vi "testAttitude.vi"() -> ()   [LabVIEW 2011]
uses:
  Instance           3 20Saved   testAttitude .vi
  Instance           1 20Saved   testAttitude .vi
  Instance           2 20Saved   testAttitude .vi
  sbgLabView/sbgLabView.lvlib
panel:
  out "triggerMask":string
  out "XY Graph":cluster{"Y":dbl[], "Y":dbl[]}[](graph)
  out "yaw":sgl format="%#.2f"
  out "pitch":sgl format="%#.2f"
  out "roll":sgl format="%#.2f"
  in  "stop main loop":bool
  in  "Com Port":string
  in  "BaudRate":dbl
  # "sbgLabView Example, Display euler angles for IG devices, Version 1.1"
  # "Copyright (C) SBG Systems 2007-2012 - All right reserved."
  # "www.sbg-systems.com"
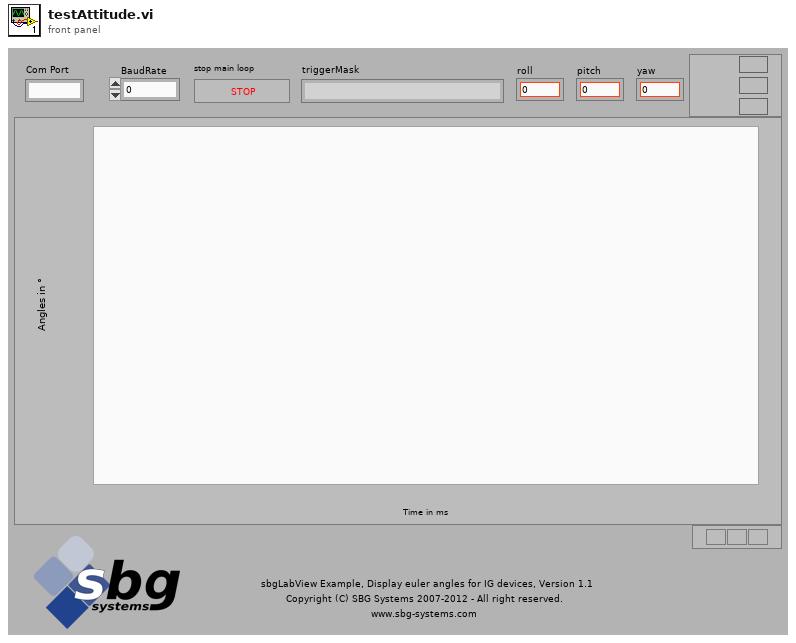
[diagram p1: front panel]
types:
  T1 = cluster{"q0":sgl, "q1":sgl, "q2":sgl, "q3":sgl, "roll":sgl, "pitch":sgl, "yaw":sgl, "ma0":sgl, "ma1":sgl, "ma2":sgl, "ma3":sgl, "ma4":sgl, "ma5":sgl, "ma6":sgl, "ma7":sgl, "ma8":sgl, "g0":sgl, "g1":sgl, "g2":sgl, "a0":sgl, "a1":sgl, "a2":sgl, "m0":sgl, "m1":sgl, "m2":sgl, "t0":sgl, "t1":sgl, "gT0":sgl, "gT1":sgl, "gT2":sgl, "gR0":u16, "gR1":u16, "gR2":u16, "aR0":u16, "aR1":u16, "aR2":u16, "mR0":u16, "mR1":u16, "mR2":u16, "tR0":u16, "tR1":u16, "gTR0":u16, "gTR1":u16, "gTR2":u16, "timeSinceReset":u32, "deviceStatus":sgl, "@dummy control@":u32, "gpsLatitude":dbl, "gpsLongitude":dbl, "gpsAltitude":i32, "gpsV0":i32, "gpsV1":i32, "gpsV2":i32, "gpsHeading":sgl, "gpsHorAccuracy":u32, "gpsVertAccuracy":u32, "gpsSpeedAccuracy":u32, "gpsHeadingAccuracy":sgl, "gpsTimeMs":u32, "gpsFlags":u8, "gpsNbSats":u8, "@dummy control@":u16, "gpsTrueHeading":sgl, "gpsTrueHeadingAccuracy":sgl, "baroPressure":sgl, "baroAltitude":sgl, "@dummy control@":u32, "p0":dbl, "p1":dbl, "p2":dbl, "v0":sgl, "v1":sgl, "v2":sgl, "attitudeAccuracy":sgl, "positionAccuracy":sgl, "velocityAccuracy":sgl, "utcYear":u8, "utcMonth":sgl, "utcDay":sgl, "utcHour":sgl, "utcMin":sgl, "utcSec":u8, "@dummy control@":u16, "utcNano":u32, "magCalibData0":u32, "magCalibData1":u32, "magCalibData2":u32, "odoRawVel0":sgl, "odoRawVel1":sgl, "deltaAngleX":sgl, "deltaAngleY":sgl, "deltaAngleZ":sgl, "heave":sgl}
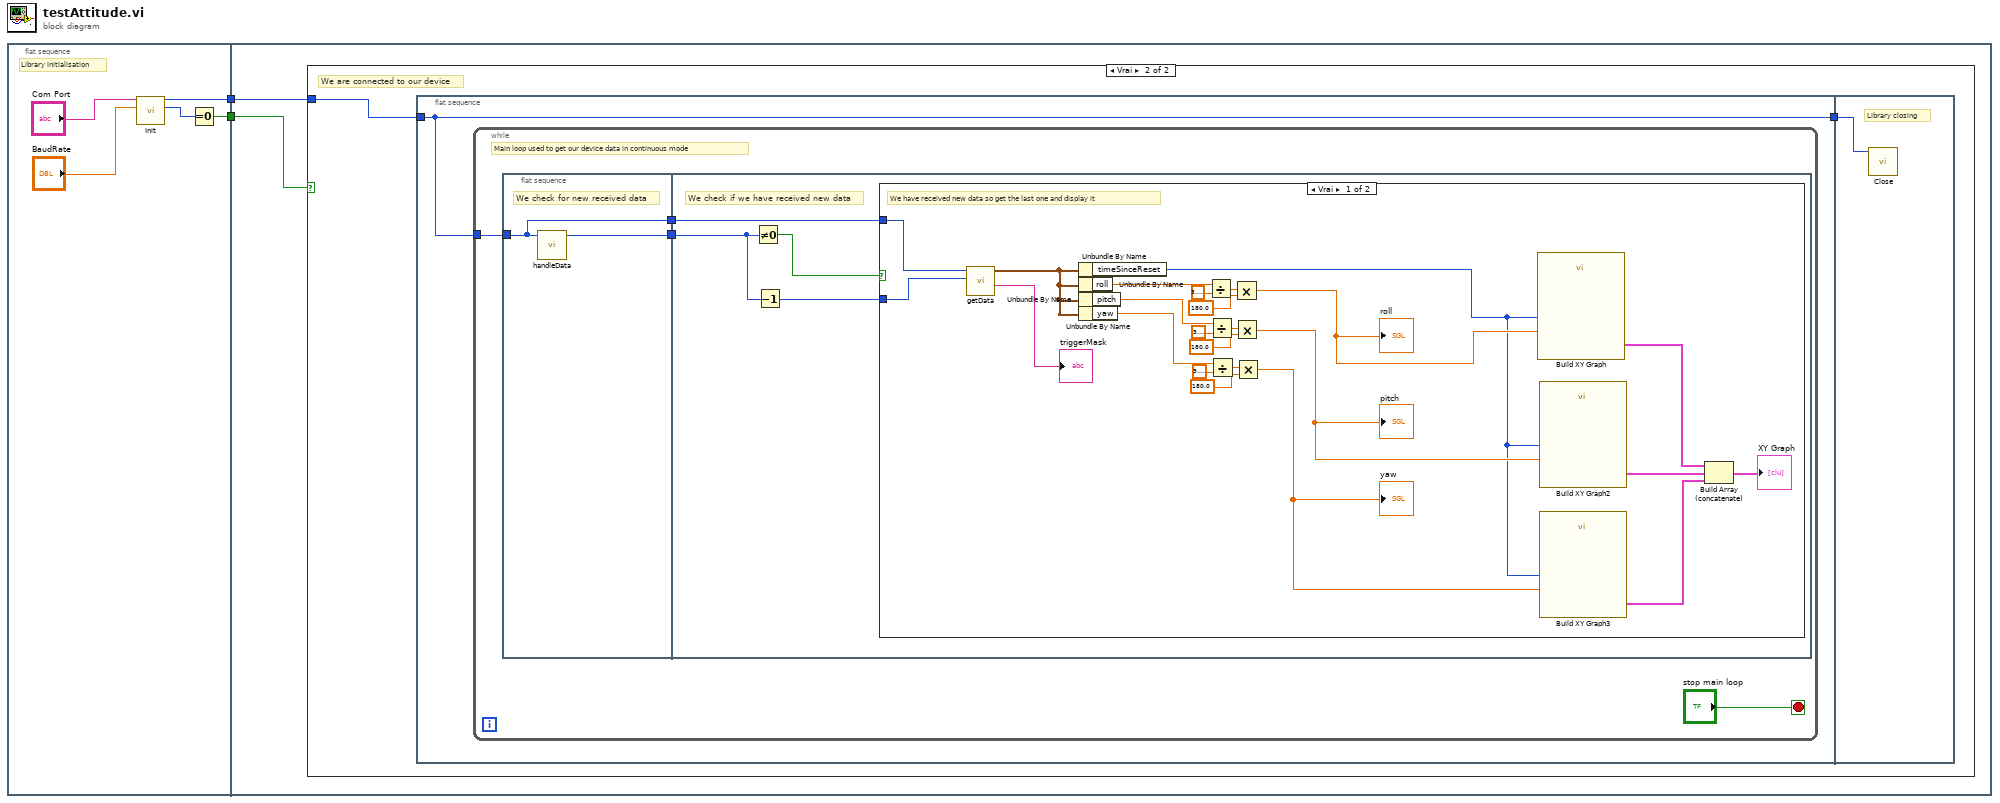
[diagram p0: block diagram]
diagram:
  n1 = flat-sequence {
    tunnel: [w5] -> w2
    tunnel: [w3] -> w1
    tunnel: w2 -> [w8]
    tunnel: w1 -> [w9]
    frame #0 {
      # "Library initialisation"
      n2 = call "Init.vi"("baudRate"="BaudRate", "deviceName"="Com Port") -> ("return type"=w4:i32, "pHandle"=w5:u32)  [unwired: 7 in, 1 out]
      n3 = Equal To 0?(x=w4) -> (x = 0?=w3:bool)
    }
    frame #1 {
      n4 = case shown="Vrai" w9 {
        tunnel: w8 -> [_ w11]
        frame False {
          # "We are not connected to our device"
        }
        frame True {
          # "We are connected to our device"
          n5 = flat-sequence {
            tunnel: w11 -> [w12]
            tunnel: [w12] -> w10
            tunnel: w10 -> [w47]
            frame #0 {
              n6 = while {
                tunnel: w12 -> [w16]
                stop <- "stop main loop" stop-if-true
                # "Main loop used to get our device data in continuous mode"
                n7 = flat-sequence {
                  tunnel: w16 -> [w17]
                  tunnel: [w18] -> w14
                  tunnel: [w17] -> w13
                  tunnel: w14 -> [w21]
                  tunnel: w13 -> [w19]
                  frame #0 {
                    # "We check for new received data"
                    n8 = call "handleData.vi"("pHandle"=w17) -> ("pNumData"=w18:u32)  [unwired: 8 in, 2 out]
                  }
                  frame #1 {
                    # "We check if we have received new data"
                    n9 = Not Equal To 0?(x=w21) -> (x != 0?=w22:bool)
                    n10 = Decrement(x=w21) -> (x-1=w20:u32)
                    n11 = case shown="Vrai" w22 {
                      tunnel: w20 -> [w26 _]
                      tunnel: w19 -> [w25 _]
                      frame True {
                        # "We have received new data so get the last one and display it"
                        n12 = call "getData.vi"("index"=w26, "pHandle"=w25) -> ("triggerMask"=→"triggerMask":string, "pData"=w46:T1)  [unwired: 6 in, 2 out]
                        n13 = Unbundle By Name(w46) -> ("timeSinceReset"=w24:u32)
                        n14 = Unbundle By Name(w46) -> ("roll"=w39:sgl)
                        n15 = Unbundle By Name(w46) -> ("pitch"=w31:sgl)
                        n16 = Unbundle By Name(w46) -> ("yaw"=w30:sgl)
                        n17 = Divide(x=w39, y=3.141592653589793) -> (x/y=w41:dbl)
                        n18 = Divide(x=w31, y=3.141592653589793) -> (x/y=w37:dbl)
                        n19 = Divide(x=w30, y=3.141592653589793) -> (x/y=w34:dbl)
                        n20 = Multiply(x=w41, y=180.0) -> (x*y=w29:dbl)
                        "roll" <- w29
                        n21 = Multiply(x=w37, y=180.0) -> (x*y=w28:dbl)
                        "pitch" <- w28
                        n22 = Multiply(x=w34, y=180.0) -> (x*y=w27:dbl)
                        "yaw" <- w27
                        n23 = call "Build XY Graph"("Y Input"=w29, "X Input"=w24) -> ("XY Graph"=w45:cluster{"Y":dbl[], "Y":dbl[]}[])  [unwired: 8 in, 1 out]
                        n24 = call "Build XY Graph2"("Y Input"=w28, "X Input"=w24) -> ("XY Graph"=w44:cluster{"Y":dbl[], "Y":dbl[]}[])  [unwired: 8 in, 1 out]
                        n25 = call "Build XY Graph3"("Y Input"=w27, "X Input"=w24) -> ("XY Graph"=w42:cluster{"Y":dbl[], "Y":dbl[]}[])  [unwired: 8 in, 1 out]
                        n26 = Build Array (concatenate)(w45, w44, w42) -> (→"XY Graph":cluster{"Y":dbl[], "Y":dbl[]}[])
                      }
                      frame False {
                        # "No new data received"
                      }
                    }
                  }
                }
              }
            }
            frame #1 {
              # "Library closing"
              n27 = call "Close.vi"("pHandle"=w47) -> ()  [unwired: 9 in, 2 out]
            }
          }
        }
      }
    }
  }
